vi "HighSpeedEServerIsConnected.vi"(9 "HighSpeedEServer":refnum<k24>, 11 "error in (no error)":errorcluster) -> (1 "Connected":bool, 3 "error out":errorcluster)   [LabVIEW 2015, in "UnderAutomation.Yaskawa.lvlib"]
uses:
  UnderAutomation.Yaskawa.lvlib
  C:/Users/fg/Documents/Yaskawa.vi/LabVIEW_2024/UnderAutomation.Yaskawa/lib/UnderAutomation.Yaskawa.dll
  LabVIEW_2024/UnderAutomation.Yaskawa/lib/UnderAutomation.Yaskawa.dll
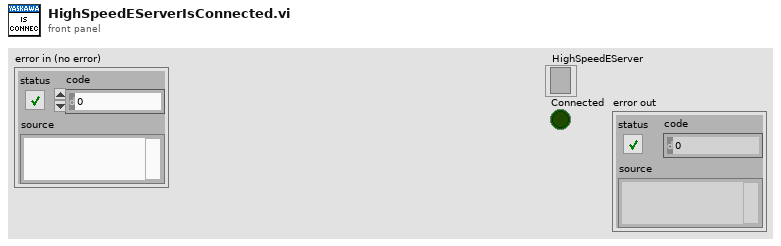
[diagram p1: front panel]
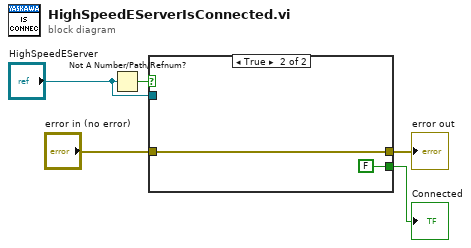
[diagram p0: block diagram]
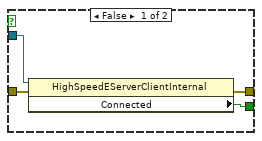
[diagram p2: hidden frame]
diagram:
  n1 = Not A Number/Path/Refnum?(number/path/refnum="HighSpeedEServer") -> (NaN/Path/Refnum?=w2:bool)
  n2 = case shown="True" w2 {
    tunnel: "HighSpeedEServer" -> [w9 _]
    tunnel: "error in (no error)" -> [w8 w11]
    tunnel: [w7 FALSE ("Connected")] -> w4
    tunnel: [w6 w11] -> w3
    frame False {
      n3 = property class="HighSpeedEServerClientInternal"(reference=w9, error in=w8) -> (error out=w6:errorcluster, "Connected"=w7:bool)  [unwired: 1 out]
    }
    frame True {
    }
  }
  "Connected" <- w4
  "error out" <- w3
